vi "Automotive ECU - Steering Control.vi"() -> ()   [LabVIEW 2013]
doc: "Sample numeric display item."
uses:
  <vilib>/NI Veristand/Display Template Support/Display Template Support.llb/cluster_Screen Item Settings.ctl
  <vilib>/NI Veristand/Display Template Support/Display Template Support.llb/cluster_Graph Scale Settings.ctl
  <vilib>/NI Veristand/Display Template Support/Display Template Support.llb/cluster_Graph Plot Settings.ctl
  NationalInstruments.VeriStand.SystemStorage
  <vilib>/NI Veristand/Display Template Support/Display Template Support.llb/enum_Display Template Handler Minimal To Widget Msg.ctl
  <vilib>/NI Veristand/Display Template Support/Display Template Support.llb/enum_Display Template Handler Minimal To Workspace.ctl
  Support/Slide Parameters.ctl
  Support/PWM Object Parameters.ctl
  <vilib>/NI Veristand/Execution/Workspace/NI VeriStand - Get Single Channel Value.vi
  <vilib>/NI Veristand/Execution/Workspace/NI_VS Workspace ExecutionAPI.lvlib
panel:
  in  "Slide":dbl(slide)=0.5 min=0.0 max=100.0 step=0.01 scale=0.1..0.9 scale format="%#5.2g"
  out "Label":string="Numeric"
  in  "NIVS.System Definition Root":refnum<k24>
  in  "NIVS.Gateway IP Address":string
  in  "Item.Data":T1
  # "RIGHT"
  # "LEFT"
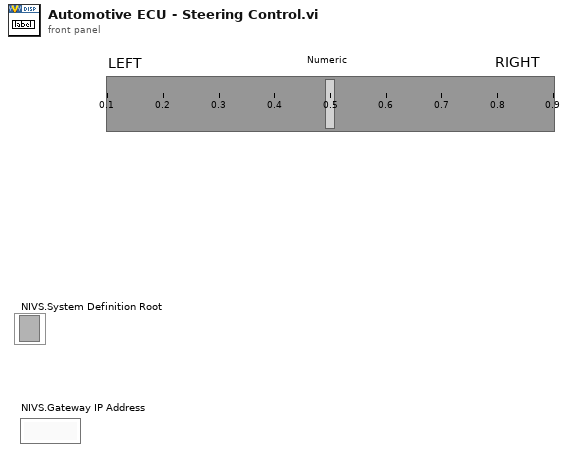
[diagram p1: front panel]
types:
  T1 = typedef "cluster_Screen Item Settings.ctl" = cluster{"Template VI":string, "Position X":i32, "Position Y":i32, "Custom":string, "Show Title Bar":bool, "ID":i32, "Always On Top":bool, "Allow Resize":bool, "Allow Minimize":bool, "Allow Close":bool, "Size to Screen":bool, "Screen.ID":i32, "State":enum16{"Normal", "New"}, "Title":string, "Window Bounds":cluster{"[0]":i16, "[1]":i16, "[2]":i16, "[3]":i16}, "Channel Ref":u64, "Unit":string, "Default Units?":bool, "Flash Limit?":bool, "Color 1":u32, "Color 2":u32, "Color 3":u32, "Color 4":u32, "Bck Color":u32, "Fore Color":u32, "Limit 1":dbl, "Limit 2":dbl, "Limit 3":dbl, "Limit 4":dbl, "Limit Mode 1":i32, "Limit Mode 2":i32, "Limit Mode 3":i32, "Limit Mode 4":i32, "Scale Precision":i32, "Scale Min":dbl, "Scale Max":dbl, "Format":i32, "Precision":i32, "Background Type":i32, "IDs":i32[], "Units":string[], "Labels":string[], "Scale Factor":dbl, "Scale Offset":dbl, "YScale Index":u32[], "XScale":T2, "YScales":T2[], "Plots":T3[], "Update Period":dbl, "History Length":dbl, "My.Ref":refnum<vi>, "Is Control?":bool, "Channel Paths":string[], "Custom Data":variant}
  T2 = typedef "cluster_Graph Scale Settings.ctl" = cluster{"Format":u8, "Precision":u8, "Fit":u8, "Label":string, "Use Default Label":bool, "Label Visible":bool, "Min":dbl, "Max":dbl}
  T3 = typedef "cluster_Graph Plot Settings.ctl" = cluster{"Bar Style":u8, "Fill To":i16, "Fill/PtColor":u32, "Line Style":u8, "Line Width":u8, "Color":u32, "Interp":u8, "Point Style":u8}
  T4 = typedef "enum_Display Template Handler Minimal To Workspace.ctl" = cluster{"Operation":enum16{"SetCustomData", "DeleteItem"}, "Data":variant}
  T5 = typedef "enum_Display Template Handler Minimal To Widget Msg.ctl" = enum16{"Stop", "LaunchConfigDialog"}
  T6 = typedef "Slide Parameters.ctl" = cluster{"Data cluster in":T7, "BG color":u32, "Initialized?":bool, "PWM Rails":dbl[], "Default Control Values":variant[]}
  T7 = typedef "PWM Object Parameters.ctl" = cluster{"RIO?":bool, "Label":string, "PWM Channel Path":cluster{"NodePathArray":string[], "Node Path":string}}
  T8 = typedef "NI_VS Workspace ExecutionAPI.lvlib/WorkspaceAPI.ctl" = refnum<k24>
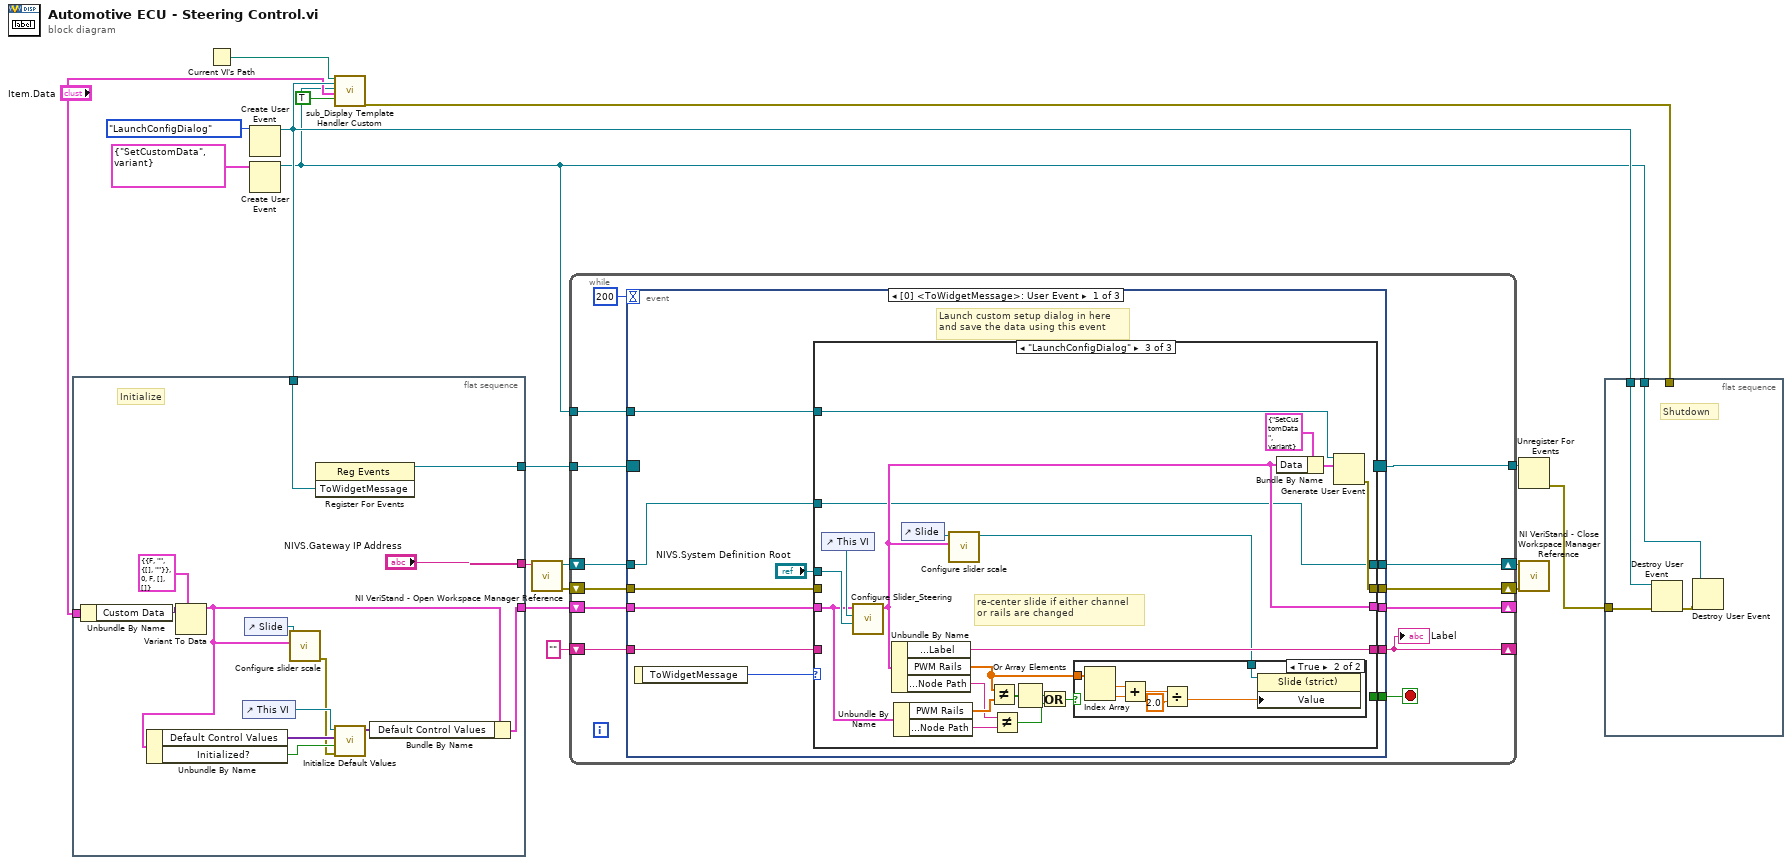
[diagram p0: block diagram]
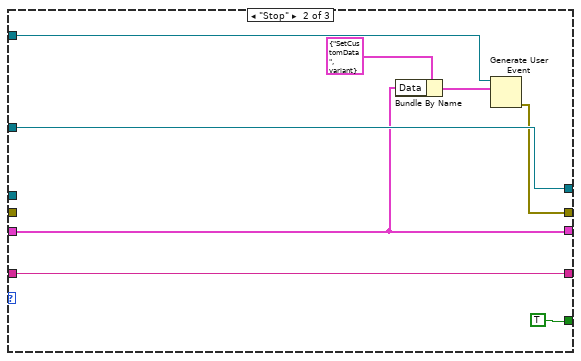
[diagram p3: hidden frame]
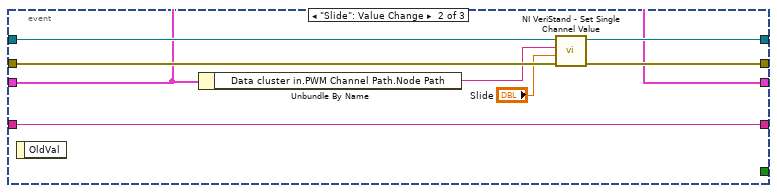
[diagram p5: hidden frame]
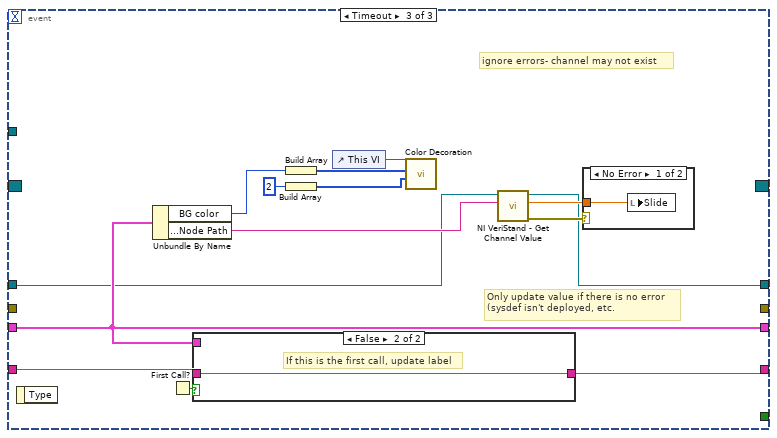
[diagram p6: hidden frame]
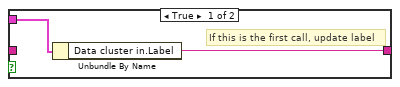
[diagram p8: hidden frame]
diagram:
  n1 = flat-sequence {
    tunnel: [w32] -> w16
    tunnel: w13 -> [w31]
    tunnel: "Item.Data" -> [w30]
    tunnel: [w20] -> w7
    tunnel: ["NIVS.Gateway IP Address"] -> w2
    frame #0 {
      # "Initialize"
      n2 = Unbundle By Name(w30) -> ("Custom Data"=w29:variant)
      n3 = Variant To Data(type=T6 {"Data cluster in"={"RIO?"=FALSE, "Label"="", "PWM Channel Path"={"NodePathArray"=[], "Node Path"=""}}, "BG color"=0, "Initialized?"=FALSE, "PWM Rails"=[], "Default Control Values"=[]} ("Slide Parameters"), Variant=w29) -> (data=w21:T6)  [unwired: 1 in, 1 out]
      n4 = Unbundle By Name(w21) -> ("Default Control Values"=w24:variant[], "Initialized?"=w22:bool)
      n5 = control-ref of="This VI"() -> (w23:refnum<vi>)
      n6 = control-ref of="Slide"() -> (w26:refnum<vi>)
      n7 = call "Configure slider scale.vi"("Slide Parameters"=w21, "Slide in"=w26) -> ("error out"=w19:errorcluster)  [unwired: 8 in, 1 out]
      n8 = register-events(w31) -> (reference out=w32:refnum<event-registration>)  [unwired: 2 in, 1 out]
      n9 = call "Initialize Default Values.vi"("error in (no error)"=w19, "Initialized?"=w22, "Default Control Values in"=w24, "VI in"=w23) -> ("Default Control Values out"=w25:variant[])  [unwired: 6 in, 1 out]
      n10 = Bundle By Name(cluster=w21, "Default Control Values"=w25) -> (w20:T6)
    }
  }
  n11 = Current VI's Path() -> (path=w11:path)
  n12 = Create User Event(user event datatype=enum_Display_Template_Handler_Minimal_To_Widget_Msg."LaunchConfigDialog" ("ToWidgetMessage")) -> (user event=w13:refnum<user-event>)  [unwired: 1 in, 1 out]
  n13 = Create User Event(user event datatype=T4 {"Operation"=enum."SetCustomData", "Data"=variant} ("Data")) -> (user event=w9:refnum<user-event>)  [unwired: 1 in, 1 out]
  n14 = call <vilib>:"sub_Display Template Handler Custom.vi"("Parent.Path"=w11, "ToWidgetEvent"=w13, "ToWorkspace"=w9, "Item.Data"="Item.Data", "Resizable"=TRUE) -> ("error out"=w18:errorcluster)  [unwired: 14 in]
  n15 = call <vilib>:"NI VeriStand - Open Workspace Manager Reference.vi"("Gateway IP Address (\"\": localhost)"=w2) -> ("error out"=w5:errorcluster, "WorkspaceManager"=w6:T8)  [unwired: 9 in]
  n16 = while {
    tunnel: w16 -> [w45]
    tunnel: [w43] -> w15
    tunnel: w9 -> [w42]
    shift-right: [w34] -> _
    shift-left: w7 -> [w41]
    shift-right: [w38] -> w4
    shift-left: w6 -> [w40]
    shift-right: [w35] -> w3
    shift-left: w5 -> [w39]
    shift-right: [w36] -> _
    shift-left: "" ("Out") -> [w37]
    stop <- w44 stop-if-true
    n17 = event shown="[0] <ToWidgetMessage>: User Event" {
      selector: w45 -> [_ _ _]
      dyn-events: [_ _ _] -> w43
      timeout: 200 -> [_ _ _]
      tunnel: [w56 _ _] -> w44
      tunnel: w42 -> [w55 _ _]
      tunnel: w41 -> [w51 w99 w111]
      tunnel: w40 -> [w54 w100 w106]
      tunnel: w39 -> [w49 w101 _]
      tunnel: [w53 w103 w105] -> w38
      tunnel: [w48 w104 _] -> w35
      tunnel: [w47 w102 w117] -> w36
      tunnel: w37 -> [w46 w102 w116]
      tunnel: [w50 w99 w111] -> w34
      event User Event {
        # "Launch custom setup dialog in here\nand save the data using this event"
        n18 = event-data() -> ("ToWidgetMessage"=w57:T5)  [unwired: 1 out]
        n19 = case shown="\"LaunchConfigDialog\"" w57 {
          tunnel: [_ TRUE _] -> w56
          tunnel: w55 -> [_ w65 w87]
          tunnel: w54 -> [w61 w68 w76]
          tunnel: [w61 w68 w76] -> w53
          tunnel: "NIVS.System Definition Root" -> [_ _ w85]
          tunnel: w51 -> [w60 w64 w79]
          tunnel: [w60 w64 w78] -> w50
          tunnel: w49 -> [w58 _ _]
          tunnel: [w58 w63 w86] -> w48
          tunnel: [w59 w62 w83] -> w47
          tunnel: w46 -> [w59 w62 _]
          frame Default {
          }
          frame "Stop" {
            n20 = Bundle By Name(cluster=T4 {"Operation"=enum."SetCustomData", "Data"=variant} ("event data"), "Data"=w64) -> (w66:T4)
            n21 = Generate User Event(user event=w65, event data cluster=w66) -> (error out=w63:errorcluster)  [unwired: 2 in, 1 out]
          }
          frame "LaunchConfigDialog" {
            # "re-center slide if either channel \nor rails are changed"
            n22 = control-ref of="This VI"() -> (w84:refnum<vi>)
            n23 = call "Configure Slider_Steering.vi"("NIVS.System Definition Root"=w85, "VI Reference"=w84, "Slide Parameters In"=w79) -> ("Slide Parameters Out"=w78:T6)  [unwired: 7 in, 1 out]
            n24 = Unbundle By Name(w78) -> ("Data cluster in.Label"=w83:string, "PWM Rails"=w77:dbl[], "Data cluster in.PWM Channel Path.Node Path"=w75:string)
            n25 = Unbundle By Name(w79) -> ("PWM Rails"=w81:dbl[], "Data cluster in.PWM Channel Path.Node Path"=w74:string)
            n26 = control-ref of="Slide"() -> (w82:refnum<vi>)
            n27 = call "Configure slider scale.vi"("Slide Parameters"=w78, "Slide in"=w82) -> ("Slide reference out"=w70:refnum<vi>)  [unwired: 8 in, 1 out]
            n28 = Not Equal?(x=w77, y=w81) -> (x != y?=w80:bool[])
            n29 = Not Equal?(x=w75, y=w74) -> (x != y?=w73:bool)
            n30 = Or Array Elements(Boolean array=w80) -> (logical OR=w71:bool)
            n31 = Or(x=w71, y=w73) -> (x .or. y?=w72:bool)
            n32 = case shown="True" w72 {
              tunnel: w77 -> [_ w94]
              tunnel: w70 -> [_ w90]
              frame False {
              }
              frame True {
                n33 = Index Array(array=w94) -> (element #1=w93:dbl, element #2=w92:dbl)  [unwired: 2 in]
                n34 = Add(x=w93, y=w92) -> (x+y=w96:dbl)
                n35 = Divide(x=w96, y=2.0) -> (x/y=w91:dbl)
                n36 = property class="Slide (strict)"(reference=w90, "Value"=w91) -> ()  [unwired: 1 in, 2 out]
              }
            }
            n37 = Bundle By Name(cluster=T4 {"Operation"=enum."SetCustomData", "Data"=variant} ("event data"), "Data"=w78) -> (w89:T4)
            n38 = Generate User Event(user event=w87, event data cluster=w89) -> (error out=w86:errorcluster)  [unwired: 2 in, 1 out]
          }
        }
      }
      event "Slide": Value Change {
        n39 = event-data() -> ()  [unwired: 2 out]
        n40 = Unbundle By Name(w99) -> ("Data cluster in.PWM Channel Path.Node Path"=w97:string)
        n41 = call <vilib>:"NI VeriStand - Set Single Channel Value.vi"("error in (no error)"=w101, "Value"="Slide", "Channel"=w97, "WorkspaceManager in"=w100) -> ("error out"=w104:errorcluster, "WorkspaceManager out"=w103:T8)  [unwired: 6 in]
      }
      event Timeout {
        # "Only update value if there is no error\n(sysdef isn't deployed, etc."
        # "ignore errors- channel may not exist"
        n42 = event-data() -> ()  [unwired: 2 out]
        n43 = Unbundle By Name(w111) -> ("BG color"=w110:u32, "Data cluster in.PWM Channel Path.Node Path"=w107:string)
        n44 = First Call?() -> (First Call?: T/F=w118:bool)
        n45 = case shown="False" w118 {
          tunnel: w116 -> [_ w122]
          tunnel: [w120 w122] -> w117
          tunnel: w111 -> [w121 _]
          frame True {
            # "If this is the first call, update label"
            n46 = Unbundle By Name(w121) -> ("Data cluster in.Label"=w120:string)
          }
          frame False {
            # "If this is the first call, update label"
          }
        }
        n47 = Build Array(w110) -> (w114:u32[])
        n48 = Build Array(u32 2 ("BG color")) -> (w113:u32[])
        n49 = control-ref of="This VI"() -> (w115:refnum<vi>)
        n50 = call "Color Decoration.vi"("VI reference"=w115, "Color Array"=w114, "Index Array"=w113) -> ()  [unwired: 7 in, 1 out]
        n51 = call-poly <vilib>:"NI VeriStand - Get Channel Value.vi"("Channel"=w107, "WorkspaceManager in"=w106) -> ("error out"=w109:errorcluster, "Value"=w108:dbl, "WorkspaceManager out"=w105:T8)  [unwired: 7 in]
        n52 = case shown="No Error" w109 {
          tunnel: w108 -> [w119 _]
          frame No Error {
            n53 = local write "Slide"(w119) -> ()
          }
          frame Error {
          }
        }
      }
    }
    "Label" <- w36
  }
  n54 = Unregister For Events(event registration refnum=w15) -> (error out=w14:errorcluster)  [unwired: 1 in]
  n55 = call <vilib>:"NI VeriStand - Close Workspace Manager Reference.vi"("error in (no error)"=w3, "WorkspaceManager"=w4) -> ()  [unwired: 9 in, 1 out]
  n56 = flat-sequence {
    tunnel: w18 -> [_]
    tunnel: w14 -> [w125]
    tunnel: w13 -> [w126]
    tunnel: w9 -> [w123]
    frame #0 {
      # "Shutdown"
      n57 = Destroy User Event(user event=w126, error in=w125) -> (error out=w124:errorcluster)
      n58 = Destroy User Event(user event=w123, error in=w124) -> ()  [unwired: 1 out]
    }
  }
